vi "Create Motion TA Element.vi"(8 "error in (no error)":errorcluster, 9 "Option":enum16{"Simple Move", "Start", "End"}(ring), 10 "Destination":dbl, 11 "Index":i32) -> (0 "error out":errorcluster, 3 "TriggerAction element out":T1)   [LabVIEW 2016, in "Hardware.lvlib" / "Motions.lvlib" / "Motions.lvclass"]
uses:
  <userlib>/Common Components/Hardware/Abstract System/Motions/Motions/Motions.lvclass
  <userlib>/Common Components/TriggerAction Q/TriggerAction Q/Element Data.ctl
  <userlib>/Common Components/Hardware/Abstract System/Motions/Motions/Data_Move.ctl
  <userlib>/Common Components/Hardware/Abstract System/Motions/Motions/Data_Update History Dst Q.ctl
  <userlib>/Common Components/Hardware/Abstract System/Motions/Motions/Data_Set Motion Status.ctl
  <userlib>/Common Components/TriggerAction Q/TriggerAction Q/TriggerAction Q.lvclass
  <vilib>/addons/_JKI.lib/Serialization/JSON/JKI JSON Serialization.lvlib
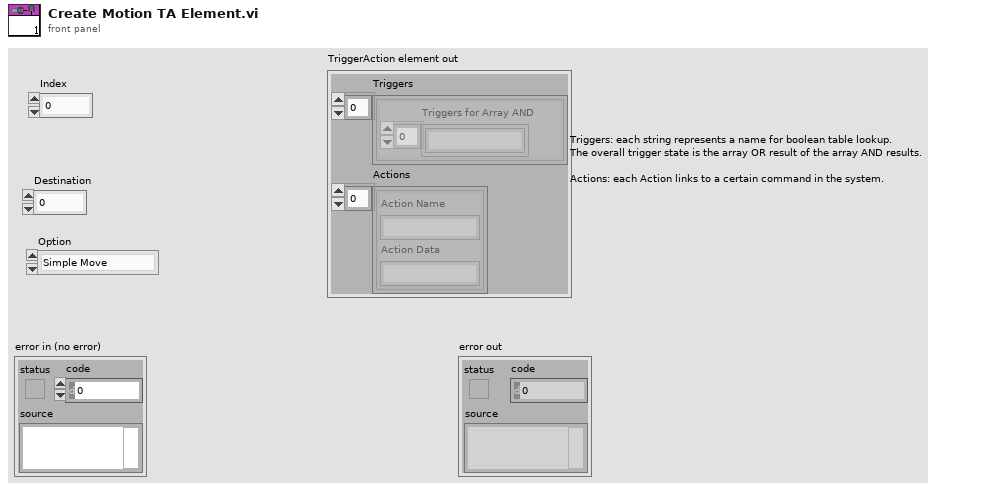
[diagram p1: front panel]
types:
  T1 = typedef "TriggerAction Q.lvclass/Element Data.ctl" = cluster{"Triggers":cluster{"Triggers for Array AND":string[]}[], "Actions":cluster{"Action Name":string, "Action Data":string}[]}
  T2 = typedef "Hardware.lvlib/Motions.lvlib/Motions.lvclass/Data_Update History Dst Q.ctl" = cluster{"Index":i32, "Destination":dbl, "Mode":enum16{"Add", "Replace"}}
  T3 = typedef "Hardware.lvlib/Motions.lvlib/Motions.lvclass/Data_Move.ctl" = cluster{"Index":i32, "Destination":dbl}
  T4 = typedef "Hardware.lvlib/Motions.lvlib/Motions.lvclass/Data_Set Motion Status.ctl" = cluster{"Index":i32, "Motion Status":bool}
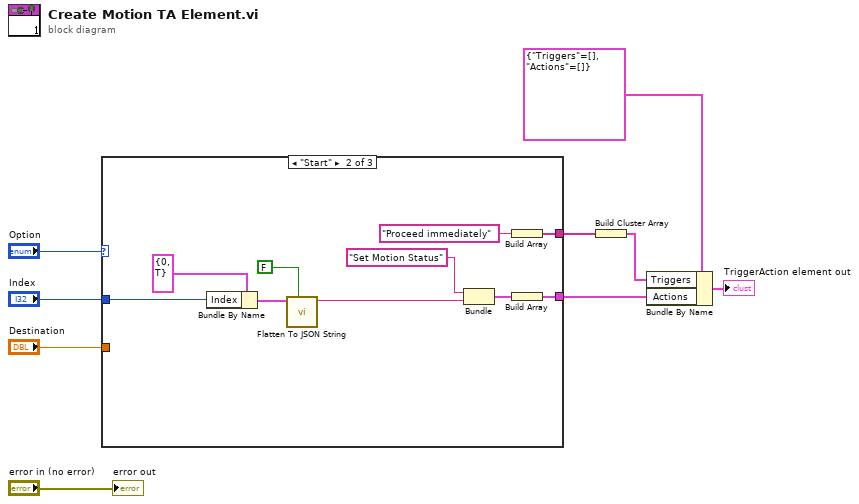
[diagram p0: block diagram]
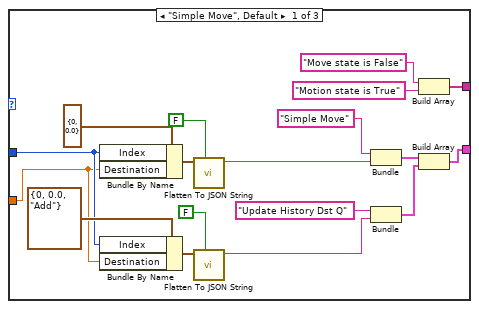
[diagram p2: hidden frame]
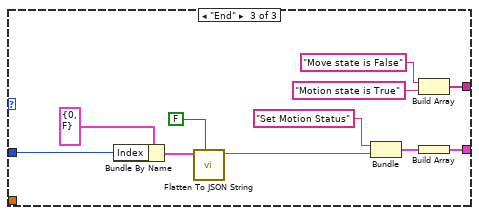
[diagram p3: hidden frame]
diagram:
  n1 = case shown="\"Start\"" "Option" {
    tunnel: "Destination" -> [w15 _ _]
    tunnel: [w22 w31 w42] -> w5
    tunnel: "Index" -> [w16 w34 w45]
    tunnel: [w12 w29 w39] -> w1
    frame "Simple Move", Default {
      n2 = Bundle By Name(cluster=T3 {"Index"=0, "Destination"=0.0} ("Set Motion Status Data cluster"), "Index"=w16, "Destination"=w15) -> (w24:T3)
      n3 = Bundle By Name(cluster=T2 {"Index"=0, "Destination"=0.0, "Mode"=enum."Add"} ("Update History Dst Q Data cluster"), "Index"=w16, "Destination"=w15) -> (w18:T2)
      n4 = call <vilib>:"Flatten To JSON String.vi"("Multiline (T)"=FALSE, "Variant"=w24) -> ("JSON String"=w27:string)  [unwired: 8 in, 1 out]
      n5 = call <vilib>:"Flatten To JSON String.vi"("Multiline (T)"=FALSE, "Variant"=w18) -> ("JSON String"=w20:string)  [unwired: 8 in, 1 out]
      n6 = Bundle("Simple Move", "JSON String"=w27) -> (w23:cluster{string, "JSON String":string})  [unwired: 1 in]
      n7 = Bundle("Update History Dst Q", "JSON String"=w20) -> (w17:cluster{string, "JSON String":string})  [unwired: 1 in]
      n8 = Build Array("Move state is False", "Motion state is True") -> (w12:string[])
      n9 = Build Array(w23, w17) -> (w22:cluster{string, "JSON String":string}[])
    }
    frame "Start" {
      n10 = Bundle By Name(cluster=T4 {"Index"=0, "Motion Status"=TRUE} ("Set Motion Status Data cluster"), "Index"=w34) -> (w33:T4)
      n11 = call <vilib>:"Flatten To JSON String.vi"("Multiline (T)"=FALSE, "Variant"=w33) -> ("JSON String"=w36:string)  [unwired: 8 in, 1 out]
      n12 = Bundle("Set Motion Status", "JSON String"=w36) -> (w32:cluster{string, "JSON String":string})  [unwired: 1 in]
      n13 = Build Array("Proceed immediately") -> (w29:string[])
      n14 = Build Array(w32) -> (w31:cluster{string, "JSON String":string}[])
    }
    frame "End" {
      n15 = Bundle By Name(cluster=T4 {"Index"=0, "Motion Status"=FALSE} ("Set Motion Status Data cluster"), "Index"=w45) -> (w44:T4)
      n16 = call <vilib>:"Flatten To JSON String.vi"("Multiline (T)"=FALSE, "Variant"=w44) -> ("JSON String"=w47:string)  [unwired: 8 in, 1 out]
      n17 = Bundle("Set Motion Status", "JSON String"=w47) -> (w43:cluster{string, "JSON String":string})  [unwired: 1 in]
      n18 = Build Array("Move state is False", "Motion state is True") -> (w39:string[])
      n19 = Build Array(w43) -> (w42:cluster{string, "JSON String":string}[])
    }
  }
  n20 = Build Cluster Array(w1) -> (w4:cluster{string[]}[])
  n21 = Bundle By Name(cluster=T1 {"Triggers"=[], "Actions"=[]} ("TriggerAction element out"), "Triggers"=w4, "Actions"=w5) -> (→"TriggerAction element out":T1)
  "error out" <- "error in (no error)"
